vi "Unpublish WS.vi"(4 "Secret ID (Default)":string, 5 "WS Name":string, 6 "Access ID (Default)":string, 8 "error in (no error)":errorcluster, 9 "Port":u16, 10 "Host":string, 11 "Scheme (HTTP)":T1) -> (0 "error out":errorcluster)   [LabVIEW 2020, in "WS Admin.lvlib"]
uses:
  WS Admin.lvlib
  Scheme.ctl
  Client Data.ctl
  HTTP Method.ctl
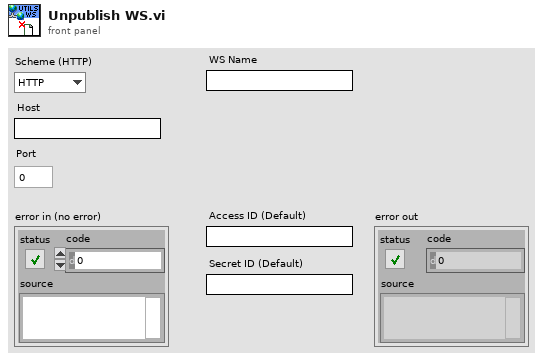
[diagram p1: front panel]
types:
  T1 = typedef "WS Admin.lvlib/Scheme.ctl" = enum16{"HTTP", "HTTPS"}
  T2 = typedef "WS Admin.lvlib/HTTP Method.ctl" = enum16{"GET", "POST", "PUT", "DELETE"}
  T3 = typedef "WS Admin.lvlib/Client Data.ctl" = cluster{"HTTP Method":T2, "URL Path":string, "Access ID":string, "Secret ID":string}
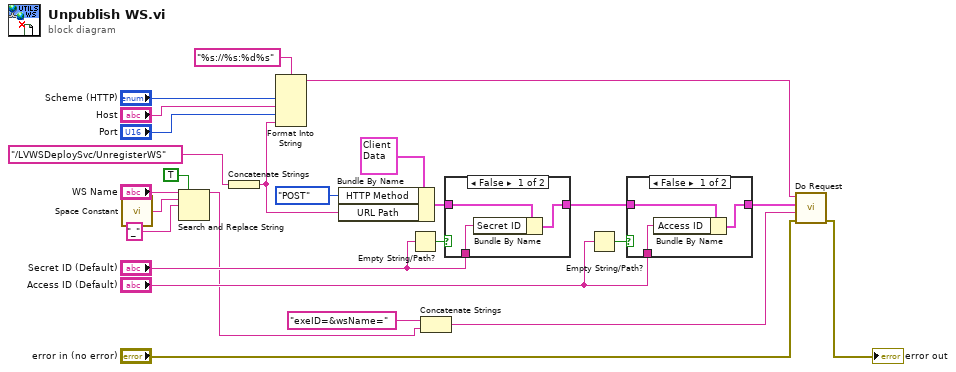
[diagram p0: block diagram]
diagram:
  n1 = call <vilib>:"Space Constant.vi"() -> ("String"=w24:string)
  n2 = Search and Replace String(replace all?=TRUE ("replace all? (F)"), input string="WS Name", search string=w24, replace string="_" ("replace string (\"\")")) -> (result string=w2:string)  [unwired: 4 in, 3 out]
  n3 = Concatenate Strings("/LVWSDeploySvc/UnregisterWS") -> (w15:string)
  n4 = Format Into String(format string="%s://%s:%d%s", "Scheme (HTTP)", "Host", "Port", w15) -> (resulting string=w5:string)  [unwired: 2 in, 1 out]
  n5 = Bundle By Name(cluster=T3 {"HTTP Method"=enum."GET", "URL Path"="", "Access ID"="PqVr/ifkAQh+lVrdPIykXlFvg12GhhQFR8H9cUhphgg=", "Secret ID"="pTe9HRlQuMfJxAG6QCGq7UvoUpJzAzWGKy5SbZ+roSU="} ("Client Data"), "HTTP Method"=HTTP_Method."POST", "URL Path"=w15) -> (w12:T3)
  n6 = Empty String/Path?(string/path="Secret ID (Default)") -> (empty?=w13:bool)
  n7 = Concatenate Strings("exeID=&wsName=", w2) -> (w1:string)
  n8 = case shown="False" w13 {
    tunnel: w12 -> [w28 w29]
    tunnel: "Secret ID (Default)" -> [w27 _]
    tunnel: [w26 w29] -> w10
    frame False {
      n9 = Bundle By Name(cluster=w28, "Secret ID"=w27) -> (w26:T3)
    }
    frame True {
    }
  }
  n10 = Empty String/Path?(string/path="Access ID (Default)") -> (empty?=w9:bool)
  n11 = case shown="False" w9 {
    tunnel: w10 -> [w32 w33]
    tunnel: "Access ID (Default)" -> [w31 _]
    tunnel: [w30 w33] -> w7
    frame False {
      n12 = Bundle By Name(cluster=w32, "Access ID"=w31) -> (w30:T3)
    }
    frame True {
    }
  }
  n13 = call "Do Request.vi"("error in (no error)"="error in (no error)", "Body (Empty)"=w1, "Client Data"=w7, "URL"=w5) -> ("error out"=→"error out":errorcluster)  [unwired: 6 in, 1 out]
